vi "Tektronix Power Supply Delay.vi"(1 "error in (no error)":errorcluster, 2 "Delay(msec)":i16) -> (0 "error out":errorcluster)   [LabVIEW 2023]
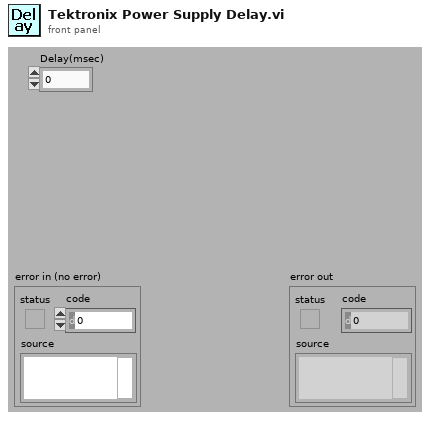
[diagram p1: front panel]
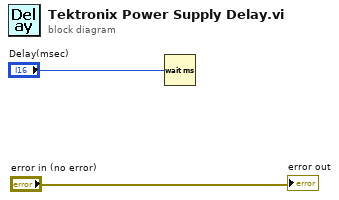
[diagram p0: block diagram]
diagram:
  n1 = Wait (ms)(milliseconds to wait="Delay(msec)") -> ()  [unwired: 1 out]
  "error out" <- "error in (no error)"
